vi "下位机.vi"() -> ()   [LabVIEW 2016]
uses:
  <vilib>/myRIO/Express VI/Onboard IO/DO/DO Express VI.xnode
  <vilib>/myRIO/Common/Instrument Driver Framework/Utilities/typedefs/Generic FPGA Reference.ctl
  <vilib>/myRIO/Common/Instrument Driver Framework/Utilities/typedefs/myRIO v1.0 Reference.ctl
  <vilib>/myRIO/Common/Instrument Driver Framework/Utilities/typedefs/Hardware Version Enum.ctl
  <vilib>/myRIO/Common/Instrument Driver Framework/Utilities/typedefs/myRIO Generic Hardware Reference.ctl
  <vilib>/myRIO/Common/Instrument Driver Framework/Utilities/vis/Is FPGA Ref Available.vi
  <vilib>/userdefined/High Color/nirio_resource_hc.ctl
  <vilib>/myRIO/Express VI/Onboard IO/PWM/PWM Express VI.xnode
  <vilib>/myRIO/Instrument Drivers/Onboard IO/PWM/vis/Set Duty Cycle and Frequency.vi
  <vilib>/myRIO/Instrument Drivers/Onboard IO/PWM/PWM.lvlib
  <vilib>/myRIO/Instrument Drivers/Onboard IO/PWM/typedefs/PWM Configuration.ctl
  <vilib>/myRIO/Common/Instrument Driver Framework/myRIO v1.0/PWM/typedefs/PWM Channels Enum.ctl
  <vilib>/myRIO/Instrument Drivers/Onboard IO/PWM/typedefs/PWM Reference.ctl
  <vilib>/myRIO/Instrument Drivers/Onboard IO/PWM/vis/myRIO PWM Open.xnode
  <vilib>/myRIO/Common/Instrument Driver Framework/myRIO v1.0/PWM/vis/myRIO v1.1 Open PWM.vi
  <vilib>/myRIO/Instrument Drivers/Onboard IO/DIO/vis/Write.vi
  <vilib>/myRIO/Instrument Drivers/Onboard IO/DIO/DIO.lvlib
  <vilib>/myRIO/Common/Instrument Driver Framework/myRIO v1.0/DIO/typedefs/DIO Channels Enum.ctl
  <vilib>/myRIO/Common/Instrument Driver Framework/myRIO v1.0/DIO/typedefs/DIO Channels List.ctl
  <vilib>/myRIO/Instrument Drivers/Onboard IO/DIO/typedefs/DIO Reference.ctl
  <vilib>/myRIO/Instrument Drivers/Onboard IO/DIO/vis/myRIO DIO Open.xnode
  <vilib>/myRIO/Common/Instrument Driver Framework/myRIO v1.0/DIO/vis/myRIO v1.1 Open DIO.vi
panel:
  in  "正反转控制":bool
  in  "右肘":dbl(knob) scale=0.025..0.125
  in  "右肩":dbl(knob) scale=0.025..0.125
  in  "右手":dbl(knob) scale=0.025..0.125
  in  "左手":dbl(knob) scale=0.025..0.125
  in  "左肘":dbl(knob) scale=0.025..0.125
  in  "左肩":dbl(knob) scale=0.025..0.125
  in  "停止按钮":bool
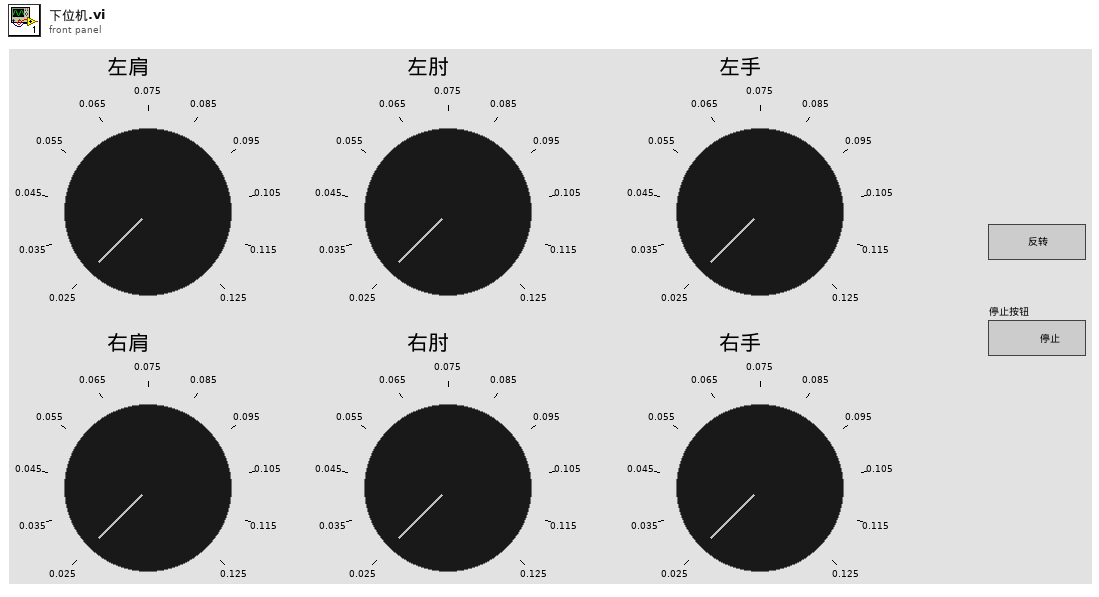
[diagram p1: front panel]
types:
  T1 = typedef "PWM.lvlib/PWM Reference.ctl" = cluster{"myRIO Reference":T2, "PWM Channels Enum":T6, "PWM Configuration":T7}
  T2 = typedef "myRIO Generic Hardware Reference.ctl" = cluster{"myRIO Model":T3, "myRIO Hardware Reference":T4}
  T3 = typedef "Hardware Version Enum.ctl" = enum16{"Unknown", "myRIO-1900", "myRIO-1950", "roboRIO", "NI ELVIS RIO CM"}
  T4 = typedef "myRIO v1.0 Reference.ctl" = cluster{"Generic FPGA Reference":T5, "Allow multiple opens":bool}
  T5 = typedef "Generic FPGA Reference.ctl" = refnum<k20>
  T6 = typedef "PWM Channels Enum.ctl" = enum16{"Not Connected", "C/PWM0", "C/PWM1", "A/PWM0", "A/PWM1", "A/PWM2", "B/PWM0", "B/PWM1", "B/PWM2", "PWM/PWM0", "PWM/PWM1", "PWM/PWM2", "PWM/PWM3", "PWM/PWM4", "PWM/PWM5", "PWM/PWM6", "PWM/PWM7", "PWM/PWM8", "PWM/PWM9"}
  T7 = typedef "PWM.lvlib/PWM Configuration.ctl" = cluster{"Frequency":dbl, "Duty Cycle":dbl}
  T8 = typedef "nirio_resource_hc.ctl" = tag
  T9 = typedef "DIO.lvlib/DIO Reference.ctl" = cluster{"myRIO Reference":T2, "DIO Channels List":T10}
  T10 = typedef "DIO Channels List.ctl" = T11[]
  T11 = typedef "DIO Channels Enum.ctl" = enum16{"Not Connected", "C/DIO0", "C/DIO1", "C/DIO2", "C/DIO3", "C/DIO4", "C/DIO5", "C/DIO6", "C/DIO7", "A/DIO0", "A/DIO1", "A/DIO2", "A/DIO3", "A/DIO4", "A/DIO5", "A/DIO6", "A/DIO7", "A/DIO8", "A/DIO9", "A/DIO10", "A/DIO11", "A/DIO12", "A/DIO13", "A/DIO14", "A/DIO15", "B/DIO0", "B/DIO1", "B/DIO2", "B/DIO3", "B/DIO4", "B/DIO5", "B/DIO6", "B/DIO7", "B/DIO8", "B/DIO9", "B/DIO10", "B/DIO11", "B/DIO12", "B/DIO13", "B/DIO14", "B/DIO15", "LED0", "LED1", "LED2", "LED3", "Button0", "DIO/DIO0", "DIO/DIO1", "DIO/DIO2", "DIO/DIO3", "DIO/DIO4", "DIO/DIO5", "DIO/DIO6", "DIO/DIO7", "DIO/DIO8", "DIO/DIO9", "SPI/CS0", "SPI/CS1", "SPI/CS2", "SPI/CS3", "LED RADIO (Green)", "LED RADIO (Red)", "LED COMM (Green)", "LED COMM (Red)", "LED MODE (Green)", "LED MODE (Red)"}
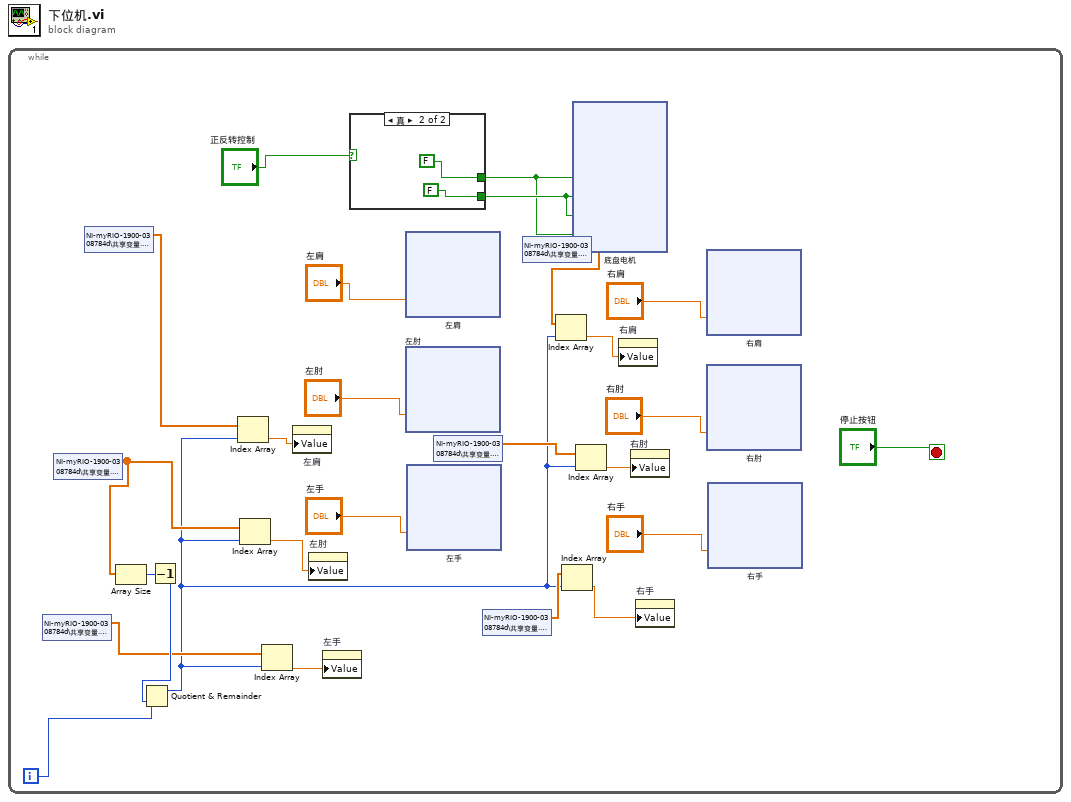
[diagram p0: block diagram]
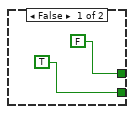
[diagram p2: hidden frame]
diagram:
  n1 = while {
    i -> [w25]
    stop <- "停止按钮" stop-if-true
    n2 = shared-variable "NI-myRIO-1900-0308784d\\共享变量.lvlib\\左手"() -> (w7:dbl[])  [unwired: 1 in, 1 out]
    n3 = shared-variable "NI-myRIO-1900-0308784d\\共享变量.lvlib\\左肘"() -> (w24:dbl[])  [unwired: 1 in, 1 out]
    n4 = shared-variable "NI-myRIO-1900-0308784d\\共享变量.lvlib\\左肩"() -> (w15:dbl[])  [unwired: 1 in, 1 out]
    n5 = Array Size(array=w24) -> (size(s)=w23:i32)
    n6 = Decrement(x=w23) -> (x-1=w22:i32)
    n7 = Quotient & Remainder(x=w25, y=w22) -> (x-y*floor(x/y)=w6:i32)  [unwired: 1 out]
    n8 = Index Array(array=w15, index=w6) -> (element=w14:dbl)
    n9 = Index Array(array=w24, index=w6) -> (element=w1:dbl)
    n10 = Index Array(array=w7, index=w6) -> (element=w5:dbl)
    n11 = property on="左肩" class="Knob (严格)"("Value"=w14) -> ()  [unwired: 2 in, 2 out]
    n12 = property on="左肘" class="Knob (严格)"("Value"=w1) -> ()  [unwired: 2 in, 2 out]
    n13 = property on="左手" class="Knob (严格)"("Value"=w5) -> ()  [unwired: 2 in, 2 out]
    n14 = case shown="真" "正反转控制" {
      tunnel: [FALSE FALSE] -> w2
      tunnel: [TRUE FALSE] -> w3
      frame False {
      }
      frame True {
      }
    }
    n15 = xnode "左肩"("Duty Cycle"="左肩") -> ()  [unwired: 1 in, 1 out]
    n16 = xnode "左肘"("Duty Cycle"="左肘") -> ()  [unwired: 1 in, 1 out]
    n17 = xnode "左手"("Duty Cycle"="左手") -> ()  [unwired: 1 in, 1 out]
    n18 = shared-variable "NI-myRIO-1900-0308784d\\共享变量.lvlib\\右肘"() -> (w13:dbl[])  [unwired: 1 in, 1 out]
    n19 = shared-variable "NI-myRIO-1900-0308784d\\共享变量.lvlib\\右手"() -> (w12:dbl[])  [unwired: 1 in, 1 out]
    n20 = shared-variable "NI-myRIO-1900-0308784d\\共享变量.lvlib\\右肩"() -> (w9:dbl[])  [unwired: 1 in, 1 out]
    n21 = Index Array(array=w9, index=w6) -> (element=w8:dbl)
    n22 = Index Array(array=w12, index=w6) -> (element=w11:dbl)
    n23 = xnode "底盘电机"("Left Out 1 (C/DIO0 (DIO0))"=w2, "Left Out 2 (C/DIO1 (DIO1))"=w3, "Right Out 1 (C/DIO2 (DIO2))"=w3, "Right Out 2 (C/DIO3 (DIO3))"=w2) -> ()  [unwired: 1 in, 1 out]
    n24 = Index Array(array=w13, index=w6) -> (element=w10:dbl)
    n25 = property on="右肩" class="Knob (严格)"("Value"=w8) -> ()  [unwired: 2 in, 2 out]
    n26 = property on="右肘" class="Knob (严格)"("Value"=w10) -> ()  [unwired: 2 in, 2 out]
    n27 = property on="右手" class="Knob (严格)"("Value"=w11) -> ()  [unwired: 2 in, 2 out]
    n28 = xnode "右肩"("Duty Cycle"="右肩") -> ()  [unwired: 1 in, 1 out]
    n29 = xnode "右肘"("Duty Cycle"="右肘") -> ()  [unwired: 1 in, 1 out]
    n30 = xnode "右手"("Duty Cycle"="右手") -> ()  [unwired: 1 in, 1 out]
  }
